vi "Header_DAQ2_gates.vi"(1 "String in":string) -> (0 "String out":string)   [LabVIEW 2013]
panel:
  out "Error":errorcluster
  in  "DAQ 2":cluster{dbl, string, "Output Channels":tag}[](array[cluster])=[{1.0, "", "Output Channels"="Dev3/ao0"}, {1.0, "", "Output Channels"="Dev3/ao1"}, {1.0, "", "Output Channels"="Dev2/ao2"}, {1.0, "", "Output Channels"="Dev2/ao3"}, {0.0, "", "Output Channels"=""}, {1.0, "", "Output Channels"=""}]
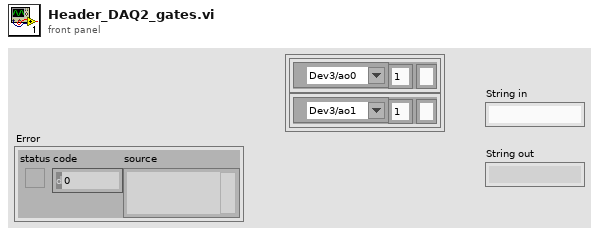
[diagram p1: front panel]
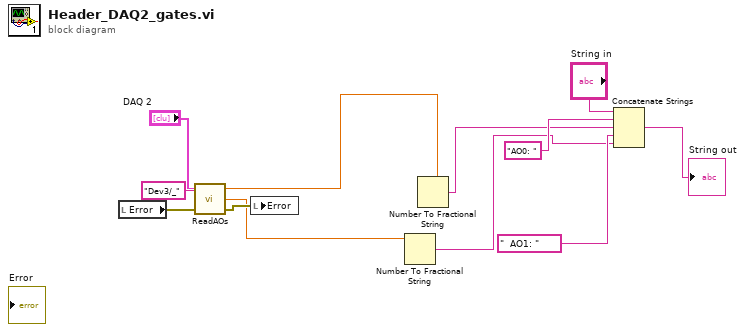
[diagram p0: block diagram]
diagram:
  n1 = local read "Error"() -> (w9:errorcluster)
  n2 = call "ReadAOs.vi"("error in"=w9, "substring (\"\")"="Dev3/_" ("substring (\"\")"), "array"="DAQ 2") -> ("error out 2"=w10:errorcluster, "AO1"=w7:dbl, "AO0"=w8:dbl)
  n3 = local write "Error"(w10) -> ()
  n4 = Number To Fractional String(number=w7) -> (F-format string=w2:string)  [unwired: 3 in]
  n5 = Number To Fractional String(number=w8) -> (F-format string=w4:string)  [unwired: 3 in]
  n6 = Concatenate Strings("String in", "AO0: ", w4, "  AO1: ", w2) -> (→"String out":string)
